vi "Connect.vi"(8 "error in":errorcluster, 11 "34980A in":refnum<class "34980A.lvclass">) -> (0 "error out":errorcluster, 3 "34980A out":refnum<class "34980A.lvclass">)   [LabVIEW 2019, in "34980A.lvlib" / "34980A.lvclass"]
uses:
  Library/34980A.lvclass
  C:/Users/Public/Documents/Development/builds/Instruments/Instruments.lvlibp/Library/Instruments.lvclass
  Library/34980A.lvclass/34980A.ctl
  builds/Instruments/Instruments.lvlibp/Accessors/Read Resource.vi
  builds/Instruments/MLTFNC.lvlibp/Library/MLTFNC.lvclass
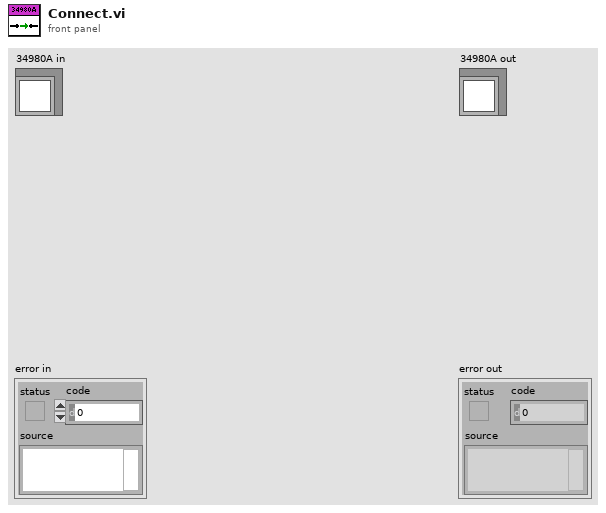
[diagram p1: front panel]
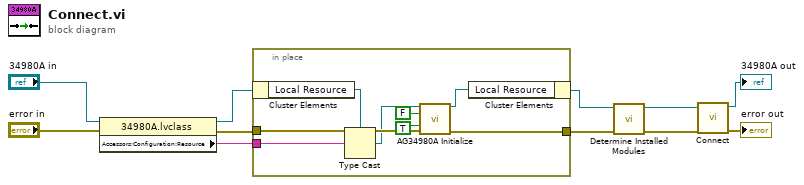
[diagram p0: block diagram]
diagram:
  n1 = property class="34980A.lvclass"(reference="34980A in", error in="error in") -> (reference out=w6:refnum<class "34980A.lvclass">, error out=w7:errorcluster, "Accessors:Configuration:Resource"=w5:string)
  n2 = in-place {
    in-place-border: w7 -> [w19]
    in-place-border: [w17] -> w3
    in-place-border: w5 -> [w16]
    n3 = in-place-cluster #1(w6) -> ("Local Resource"=w15:refnum<visa-resource-name>)
    n4 = Type Cast(type=w15, x=w16) -> (*(type *) &x=w14:refnum<visa-resource-name>)
    n5 = call <instrlib>:"AG34980A Initialize.vi"("VISA resource name"=w14, "ID Query (True)"=FALSE, "Reset (True)"=TRUE, "error in (no error)"=w19) -> ("VISA session"=w18:refnum<visa-resource-name>, "error out"=w17:errorcluster)  [unwired: 10 in]
    n6 = in-place-cluster #1("Local Resource"=w18) -> (w4:refnum<class "34980A.lvclass">)
  }
  n7 = call "Determine Installed Modules.vi"("error in"=w3, "34980A in"=w4) -> ("error out"=w2:errorcluster, "34980A out"=w1:refnum<class "34980A.lvclass">)  [unwired: 8 in]
  n8 = call-parent "Connect.vi"("error in (no error)"=w2, "MLTFNC in"=w1) -> ("error out"=→"error out":errorcluster, "MLTFNC out"=→"34980A out":refnum<class "34980A.lvclass">)  [unwired: 8 in]
